vi "WLAN - niVST - RFSA - Frequency and Level Settings.vi"(0 "instrument handle":refnum<k15>, 5 "TV Parameters(DataType)":T2 {"Standard" items=["80211A/G/J/P OFDM", "80211B/G DSSS", "80211G DSSSOFDM", "80211N MIMOOFDM", "80211AC MIMOOFDM"]; "OFDM Data Rate (Mbps)" items=["6", "9", "12", "18", "24", "36", "48", "54"]; "80211n PLCP Frame Format" items=["Mixed Format", "Greenfield Format"]; "FEC Coding Type" items=["BCC", "LDPC"]; "DSSS Data Rate (Mbps)" items=["1", "2", "5.5 CCK", "5.5 PBCC", "11 CCK", "11 PBCC", "22", "33"]}, 7 "PL":T1, 11 "error in":errorcluster) -> (4 "instrument handle":refnum<k15>, 15 "error out":errorcluster)   [LabVIEW 2012]
uses:
  TV/RW/Includes/WLAN - TV - RW - INC - TV_DataType_Cluster.ctl
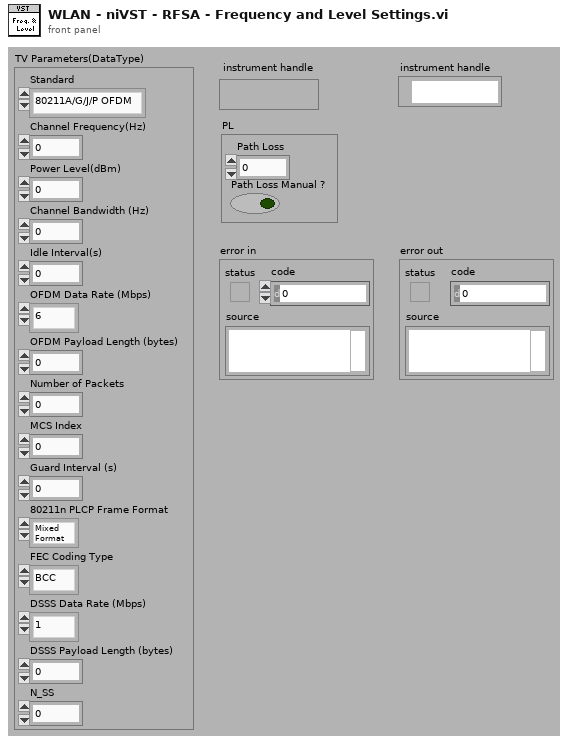
[diagram p1: front panel]
types:
  T1 = cluster{"Path Loss":dbl, "Path Loss Manual ?":bool}
  T2 = typedef "WLAN - TV - RW - INC - TV_DataType_Cluster.ctl" = cluster{"Standard":i32, "Channel Frequency(Hz)":dbl, "Power Level(dBm)":dbl, "Channel Bandwidth (Hz)":dbl, "Idle Interval(s)":dbl, "OFDM Data Rate (Mbps)":i32, "OFDM Payload Length (bytes)":i32, "Number of Packets":i32, "MCS Index":i32, "Guard Interval (s)":dbl, "80211n PLCP Frame Format":i32, "FEC Coding Type":i32, "DSSS Data Rate (Mbps)":i32, "DSSS Payload Length (bytes)":i32, "N_SS":i32}
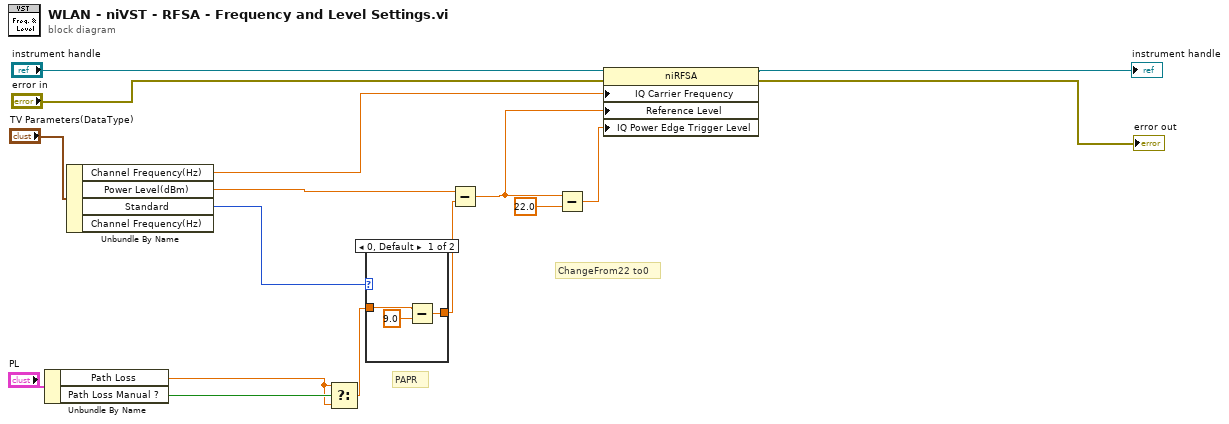
[diagram p0: block diagram]
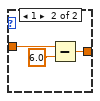
[diagram p2: hidden frame]
diagram:
  # "ChangeFrom22 to0"
  # "PAPR"
  n1 = Unbundle By Name("PL") -> ("Path Loss"=w3:dbl, "Path Loss Manual ?"=w5:bool)
  n2 = Unbundle By Name("TV Parameters(DataType)") -> ("Channel Frequency(Hz)"=w10:dbl, "Power Level(dBm)"=w9:dbl, "Standard"=w8:i32)  [unwired: 1 out]
  n3 = Select(t=w3, s=w5, f=w3) -> (s? t:f=w4:dbl)
  n4 = case shown="0, Default" w8 {
    tunnel: w4 -> [w17 w21]
    tunnel: [w19 w20] -> w7
    frame 0, Default {
      n5 = Subtract(x=w17, y=9.0) -> (x-y=w19:dbl)
    }
    frame 1 {
      n6 = Subtract(x=w21, y=6.0) -> (x-y=w20:dbl)
    }
  }
  n7 = Subtract(x=w9, y=w7) -> (x-y=w1:dbl)
  n8 = Subtract(x=w1, y=22.0) -> (x-y=w2:dbl)
  n9 = property class="niRFSA"(reference="instrument handle", error in="error in", "IQ Carrier Frequency"=w10, "Reference Level"=w1, "IQ Power Edge Trigger Level"=w2) -> (reference out=→"instrument handle":refnum<k15>, error out=→"error out":errorcluster)
